vi "Controlador.vi"(5 "x_k-2":dbl, 6 "y_k-1":dbl, 8 "x_k-1":dbl, 10 "x_k":dbl) -> (7 "y_k":dbl)   [LabVIEW 2018]
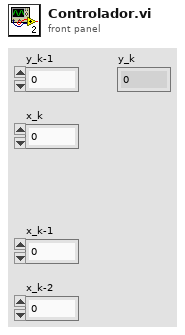
[diagram p1: front panel]
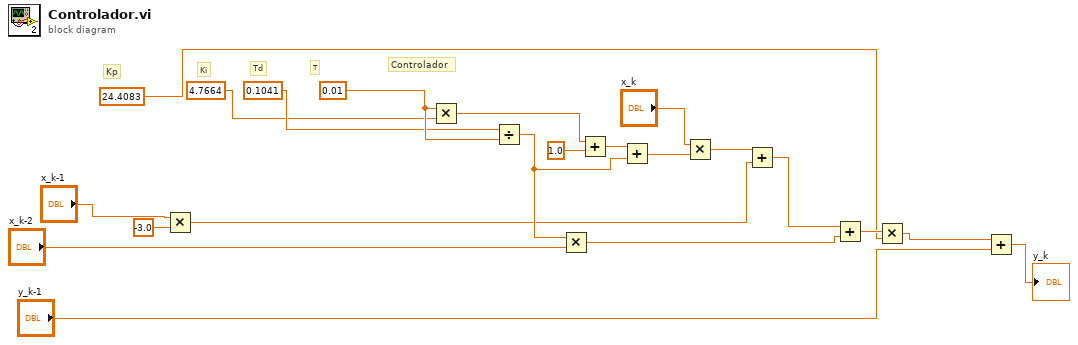
[diagram p0: block diagram]
diagram:
  w13 = 0.01
  # "Controlador"
  # "T"
  # "Td"
  # "Ki"
  # "Kp"
  n1 = Multiply(x="x_k-1", y=-3.0) -> (x*y=w5:dbl)
  n2 = Multiply(x=w13, y=4.7664) -> (x*y=w7:dbl)
  n3 = Divide(x=0.1041, y=w13) -> (x/y=w17:dbl)
  n4 = Multiply(x=w17, y="x_k-2") -> (x*y=w4:dbl)
  n5 = Add(x=w7, y=1.0 ("x")) -> (x+y=w11:dbl)
  n6 = Add(x=w11, y=w17) -> (x+y=w14:dbl)
  n7 = Multiply(x="x_k", y=w14) -> (x*y=w6:dbl)
  n8 = Add(x=w6, y=w5) -> (x+y=w19:dbl)
  n9 = Add(x=w19, y=w4) -> (x+y=w3:dbl)
  n10 = Multiply(x=w3, y=24.4083) -> (x*y=w1:dbl)
  n11 = Add(x=w1, y="y_k-1") -> (x+y=→"y_k":dbl)
